vi "Read User File Data.vi"(8 "error in":errorcluster, 10 "名称或相对路径":string, 11 "ref path":path) -> (0 "error out":errorcluster, 2 "Paramer Data":string[][](array[string]))   [LabVIEW 2017]
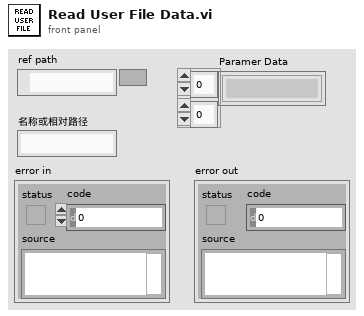
[diagram p1: front panel]
types:
  T1 = cluster{"section":string, "data type":string, "key":string[]}[]
  T2 = cluster{"Boolean":bool[], "Double":dbl[], "I32":i32[], "Path":path[], "String":string[], "U32":u32[]}[]
  T3 = cluster{"Boolean":bool[], "Double":dbl[], "I32":i32[], "Path":path[], "String":string[], "U32":u32[]}
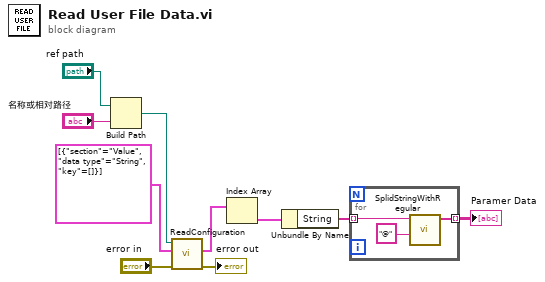
[diagram p0: block diagram]
diagram:
  n1 = Build Path(base path="ref path", name or relative path="名称或相对路径") -> (appended path=w5:path)
  n2 = call "ReadConfiguration.vi"("error in"="error in", "read config"=T1 [{"section"="Value", "data type"="String", "key"=[]}], "configuration file path"=w5) -> ("error out"=→"error out":errorcluster, "data out"=w7:T2)  [unwired: 1 in, 2 out]
  n3 = Index Array(array=w7) -> (element=w8:T3)  [unwired: 1 in]
  n4 = Unbundle By Name(w8) -> ("String"=w9:string[])
  n5 = for {
    tunnel: w9 -> [w13] mode=indexing
    tunnel: [w11] -> w10 mode=indexing
    n6 = call "SplidStringWithRegular.vi"("regular expression"="@", "String in"=w13) -> ("Array out"=w11:string[])  [unwired: 9 in]
  }
  "Paramer Data" <- w10
